vi "ReadConfig.vi"(3 "error in (no error)":errorcluster, 4 "Key":string, 5 "Section":string, 6 "Path":path) -> (0 "error out":errorcluster, 1 "Key found?":bool, 2 "Value":string)   [LabVIEW 2013]
uses:
  <vilib>/Utility/config.llb/Read Key (String).vi
  <vilib>/Utility/config.llb/NI_LVConfig.lvlib
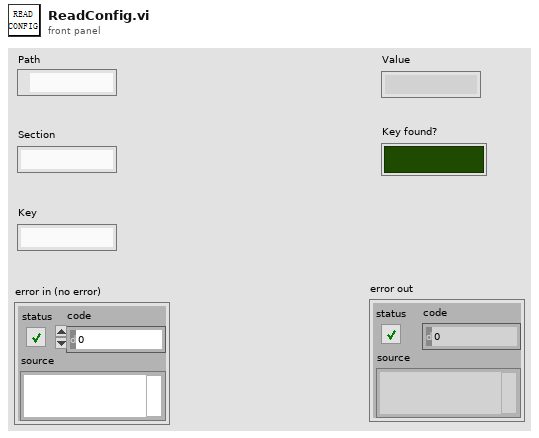
[diagram p1: front panel]
types:
  T1 = typedef "NI_LVConfig.lvlib/Config Data RefNum.ctl" = refnum<k1>
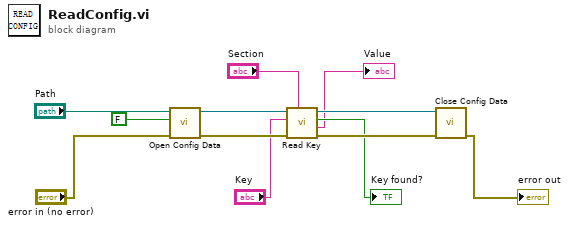
[diagram p0: block diagram]
diagram:
  n1 = call <vilib>:"Open Config Data.vi"("error in (no error)"="error in (no error)", "create file if necessary (T)"=FALSE, "configuration file path"="Path") -> ("error out"=w10:errorcluster, "refnum"=w8:T1)  [unwired: 6 in, 1 out]
  n2 = call-poly <vilib>:"Read Key.vi"("section"="Section", "error in (no error)"=w10, "key"="Key", "refnum"=w8) -> ("error out"=w9:errorcluster, "value"=→"Value":string, "found?"=→"Key found?":bool, "refnum out"=w7:T1)  [unwired: 4 in]
  n3 = call <vilib>:"Close Config Data.vi"("error in (no error)"=w9, "refnum"=w7) -> ("error out"=→"error out":errorcluster)  [unwired: 8 in, 1 out]
